vi "Project Parser_Get Files from Project.vi"(7 "To Lower Case?(T)":bool=TRUE, 8 "error in (no error)":errorcluster, 11 "Project Path":path) -> (0 "error out":errorcluster, 1 "Success?":bool, 3 "Project Files":string[](array[string]))   [LabVIEW 2019, in "Project.Dependencies Finder.lvlib"]
doc: "Extract all files from project at 'Project Path'."
uses:
  Project.Dependencies Finder.lvlib
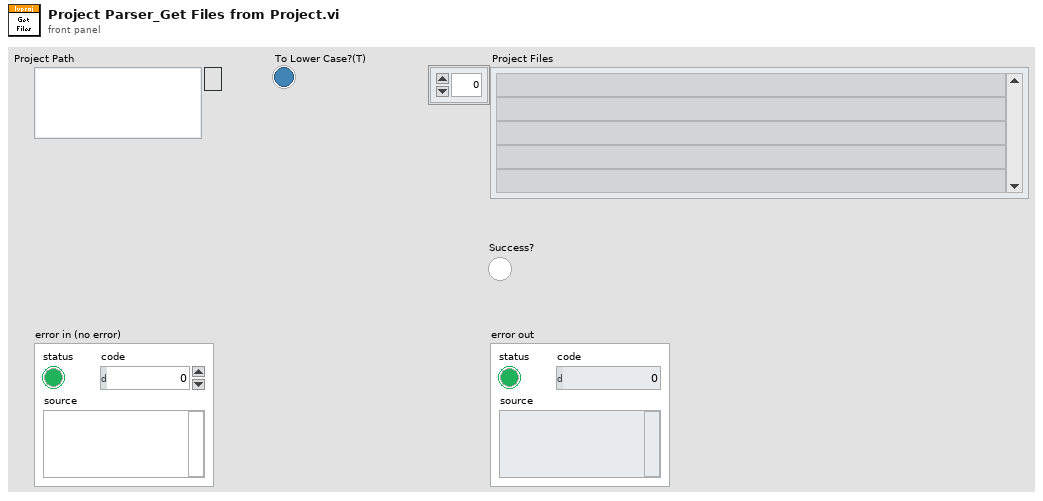
[diagram p1: front panel]
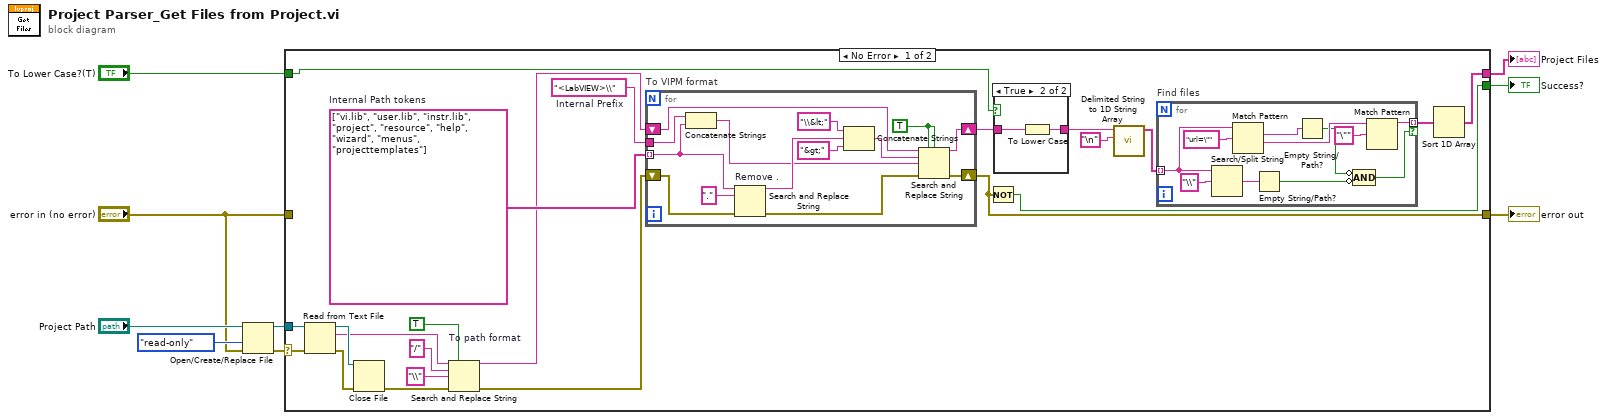
[diagram p0: block diagram]
diagram:
  n1 = Open/Create/Replace File(file path (use dialog)="Project Path", error in="error in (no error)", access (0:read/write)=enum16{"read/write", "read-only", "write-only"}."read-only") -> (refnum out=w5:refnum<file>, error out=w6:errorcluster)  [unwired: 3 in, 1 out]
  n2 = case shown="No Error" w6 {
    selector: w6 -> [w15 _]
    tunnel: [w30 _] -> w9
    tunnel: [w12 w60] -> w7
    tunnel: w5 -> [w14 _]
    tunnel: "error in (no error)" -> [_ w60]
    tunnel: [w11 _] -> w2
    tunnel: "To Lower Case?(T)" -> [w10 _]
    frame No Error {
      w29 = "<LabVIEW>\\"  # Internal Prefix
      w28 = string[] ["vi.lib", "user.lib", "instr.lib", "project", "resource", "help", "wizard", "menus", "projecttemplates"]  # Internal Path tokens
      n3 = Read from Text File(file (use dialog)=w14, error in=w15) -> (refnum out=w16:refnum<file>, text=w13:string, error out=w17:errorcluster)  [unwired: 2 in, 1 out]
      n4 = Close File(refnum=w16, error in=w17) -> (error out=w26:errorcluster)  [unwired: 1 out]
      n5 = Search and Replace String "To path format"(replace all?=TRUE ("replace all? (F)"), input string=w13, search string="/" ("String"), replace string="\\" ("replace string (\"\")"), error in=w26) -> (result string=w22:string, error out=w27:errorcluster)  [unwired: 3 in, 2 out]
      n6 = for "To VIPM format" {
        shift-right: [w47] -> w18
        shift-left: w22 -> [w48]
        shift-right: [w46] -> w12
        shift-left: w27 -> [w37]
        tunnel: w28 -> [w39] mode=indexing
        tunnel: w29 -> [w35]
        w45 = TRUE ("replace all? (F)")
        n7 = Concatenate Strings(w35, w39) -> (w38:string)
        n8 = Search and Replace String "Remove ."(input string=w39, search string="." ("String"), error in=w37) -> (result string=w43:string, error out=w36:errorcluster)  [unwired: 5 in, 2 out]
        n9 = Concatenate Strings("\\&lt;", w43, "&gt;" ("string")) -> (w40:string)
        n10 = Search and Replace String(replace all?=w45, case sensitive?=w45, input string=w48, search string=w40, replace string=w38, error in=w36) -> (result string=w47:string, error out=w46:errorcluster)  [unwired: 2 in, 2 out]
      }
      n11 = Not(x=w12) -> (.not. x?=w11:bool)
      n12 = case shown="True" w10 {
        tunnel: [w32 w34] -> w19
        tunnel: w18 -> [w32 w33]
        frame False {
        }
        frame True {
          n13 = To Lower Case(string=w33) -> (all lower case string=w34:string)
        }
      }
      n14 = call <vilib>:"Delimited String to 1D String Array.vi"("delimiter"="\n", "delimited string"=w19) -> ("string array"=w31:string[])  [unwired: 9 in]
      n15 = for "Find files" {
        tunnel: w31 -> [w55] mode=indexing
        tunnel: [w51] -> w21 mode=indexing if=w50
        n16 = Search/Split String(string=w55, search string/char (-)="\\") -> (match + rest of string=w53:string)  [unwired: 1 in, 2 out]
        n17 = Match Pattern(string=w55, regular expression="url=\"") -> (match substring=w58:string, after substring=w57:string)  [unwired: 1 in, 2 out]
        n18 = Empty String/Path?(string/path=w53) -> (empty?=w52:bool)
        n19 = Empty String/Path?(string/path=w58) -> (empty?=w56:bool)
        n20 = Compound Arithmetic op=AND(invert w56, invert w52) -> (w50:bool)
        n21 = Match Pattern(string=w57, regular expression="\"") -> (before substring=w51:string)  [unwired: 1 in, 3 out]
      }
      n22 = Sort 1D Array(array=w21) -> (sorted array=w30:string[])
    }
    frame Error {
    }
  }
  "Project Files" <- w9
  "error out" <- w7
  "Success?" <- w2
